vi "Send Generate Controller Event.vi"(7 "Priority":T1=enum."Normal" caption="Message Priority (Normal)", 8 "error in (no error)":errorcluster, 10 "Event":refnum<class "Event.lvclass">, 11 "Message Enqueuer in":refnum<class "Message Enqueuer.lvclass">) -> (0 "error out":errorcluster, 3 "Message Enqueuer out":refnum<class "Message Enqueuer.lvclass">)   [LabVIEW 2017, in "Event Actors.lvlib" / "Generate Controller Event Msg.lvclass"]
doc: "Sends the <b>Generate Controller Event Msg.lvclass</b> message.\n\nThis message will call <b>Generate Controller Event.vi</b> on the <b>Event Actors.lvlib:Controller Actor.lvclass</b> actor.\n\n<b>Generate Controller Event.vi Description</b>\nThis method generates/fires the Event wired to the input. Firing an event looks up all actors who Registered to listen to this Event and sends to them this Event on a Zero Coupling based message defined during Registration. Errors on broadcasting the event i.e. enqueuer of the registrant not existing, are ignored.\n\n<b>IMPORTANT</b> - Only call this method within actor core of your Controller Actor. From helper loops call the Send Generate Event message to self. This is to make sure your actor works with all registered listeners."
uses:
  Generate Controller Event Msg.lvclass
  <vilib>/ActorFramework/Message Enqueuer/Message Enqueuer.lvclass
  <vilib>/ActorFramework/Message Enqueuer/Message Priority.ctl
  Event/Event.lvclass
  C:/Program Files/National Instruments/LabVIEW 2017/vi.lib/ActorFramework/Message/Message.lvclass
  Generate Controller Event Msg.lvclass/Generate Controller Event Msg.ctl
  <vilib>/ActorFramework/Message Enqueuer/Message Enqueuer.lvclass/Message Enqueuer.ctl
  <vilib>/Utility/LVClass/Get LV Class Name.vi
  <resource>/AFDebug/Generate Trace for Message.vi
  <vilib>/ActorFramework/Message Priority Queue/Priority Enqueue.vi
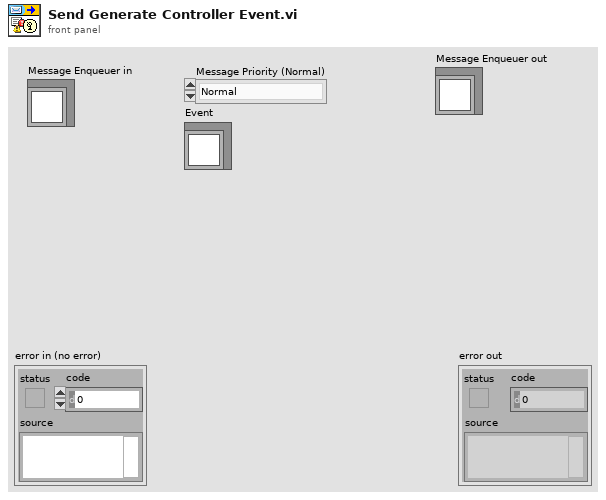
[diagram p1: front panel]
types:
  T1 = typedef "Actor Framework.lvlib/Message Enqueuer.lvclass/Message Priority.ctl" = enum16{"Low", "Normal", "High"}
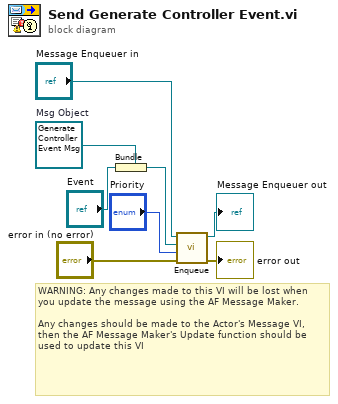
[diagram p0: block diagram]
diagram:
  w7 = refnum<class "Generate Controller Event Msg.lvclass"> refnum  # Msg Object
  # "WARNING: Any changes made to this VI will be lost when you update the message using the AF Message Maker.\n\nAny changes should be made to the Actor's Message VI, then the AF Message Maker's Update function should be used to update this VI"
  n1 = Bundle(cluster=w7, "Event") -> (w2:refnum<class "Generate Controller Event Msg.lvclass">)
  n2 = call <vilib>:"Enqueue.vi"("error in (no error)"="error in (no error)", "Message Priority (Normal)"="Priority", "Message"=w2, "Message Enqueuer in"="Message Enqueuer in") -> ("error out"=→"error out":errorcluster, "Message Enqueuer out"=→"Message Enqueuer out":refnum<class "Message Enqueuer.lvclass">)  [unwired: 6 in]
